vi "transcription.vi"() -> ()   [LabVIEW 2018]
panel:
  out "基因表达":dbl
  in  "»ùÒò¼¤·¢¿":bool
  out "产物":dbl[](array[numeric])
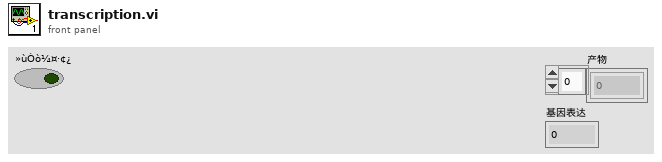
[diagram p1: front panel]
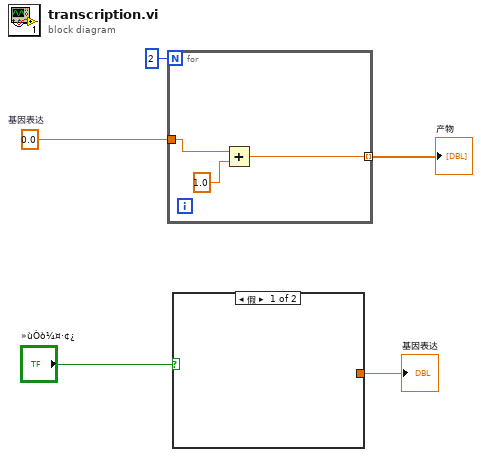
[diagram p0: block diagram]
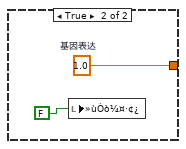
[diagram p2: hidden frame]
diagram:
  w4 = 0.0  # 基因表达
  n1 = for {
    N: 2 -> [_]
    tunnel: w4 -> [w8]
    tunnel: [w6] -> w3 mode=indexing
    n2 = Add(x=w8, y=1.0) -> (x+y=w6:dbl)
  }
  "产物" <- w3
  n3 = case shown="假" "»ùÒò¼¤·¢¿" {
    tunnel: [_ w10] -> w1
    frame False {
    }
    frame True {
      w10 = 1.0  # 基因表达
      n4 = local write "»ùÒò¼¤·¢¿"(FALSE) -> ()
    }
  }
  "基因表达" <- w1
